vi "Scan TU Number_RegExp.vi"(10 "Pattern In":string) -> (1 "OK?":bool, 3 "TU Number Out":string)   [LabVIEW 2024, in "LVarex.lvlib"]
uses:
  LVarex.lvlib
panel:
  out "First Scan?":bool
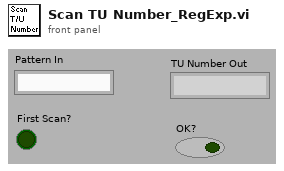
[diagram p1: front panel]
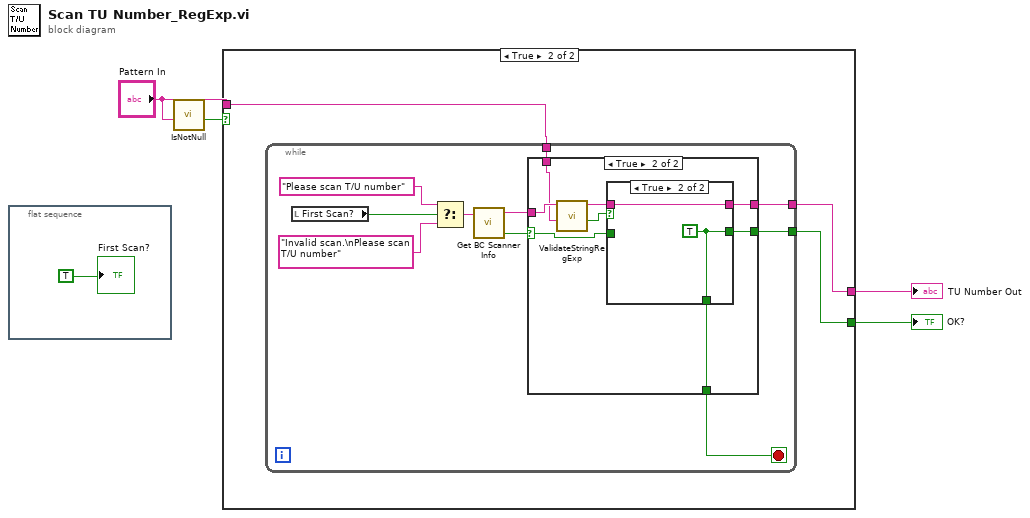
[diagram p0: block diagram]
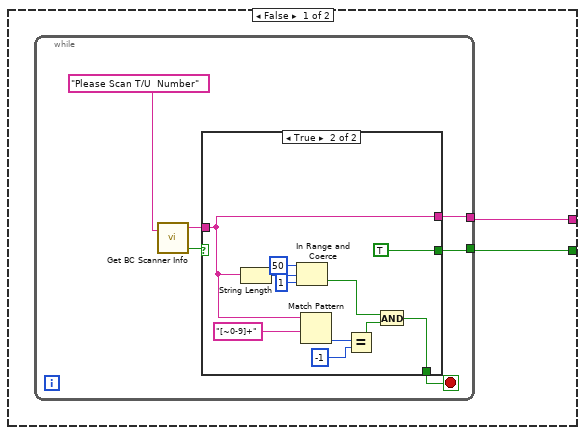
[diagram p2: hidden frame]
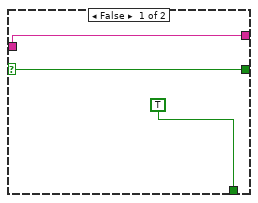
[diagram p3: hidden frame]
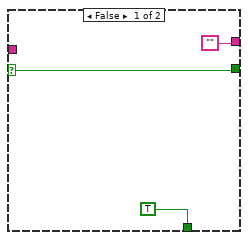
[diagram p4: hidden frame]
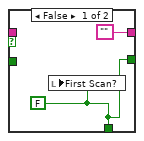
[diagram p5: hidden frame]
diagram:
  n1 = flat-sequence {
    frame #0 {
      "First Scan?" <- TRUE
    }
  }
  n2 = call "IsNotNull.vi"("String In"="Pattern In") -> ("Boolean Out"=w1:bool)  [unwired: 10 in]
  n3 = case shown="True" w1 {
    tunnel: [w7 w30] -> w4
    tunnel: [w6 w29] -> w3
    tunnel: "Pattern In" -> [_ w28]
    frame False {
      n4 = while {
        tunnel: [w11] -> w6
        tunnel: [w10] -> w7
        stop <- w9 stop-if-true
        n5 = call "Get BC Scanner Info.vi"("Prompt"="Please Scan T/U  Number") -> ("Info Out"=w8:string, "OK"=w12:bool)  [unwired: 2 in]
        n6 = case shown="True" w12 {
          selector: w12 -> [w16 _]
          tunnel: [w16 TRUE] -> w11
          tunnel: w8 -> [w15 w23]
          tunnel: [w15 w23] -> w10
          tunnel: [TRUE w17] -> w9
          frame False {
          }
          frame True {
            n7 = String Length(string=w23) -> (length=w26:i32)
            n8 = In Range and Coerce(upper limit=50, x=w26, lower limit=1) -> (In Range?=w18:bool)  [unwired: 1 out]
            n9 = Match Pattern(string=w23, regular expression="[~0-9]+") -> (offset past match=w21:i32)  [unwired: 1 in, 3 out]
            n10 = Equal?(x=w21, y=-1 ("x")) -> (x = y?=w19:bool)
            n11 = And(x=w18, y=w19) -> (x .and. y?=w17:bool)
          }
        }
      }
    }
    frame True {
      n12 = while {
        tunnel: [w34] -> w30
        tunnel: [w33] -> w29
        tunnel: w28 -> [w31]
        stop <- w32 stop-if-true
        n13 = local read "First Scan?"() -> (w38:bool)
        n14 = Select(t="Please scan T/U number", s=w38, f="Invalid scan.\nPlease scan T/U number") -> (s? t:f=w37:string)
        n15 = call "Get BC Scanner Info.vi"("Prompt"=w37) -> ("Info Out"=w36:string, "OK"=w35:bool)  [unwired: 2 in]
        n16 = case shown="True" w35 {
          selector: w35 -> [w41 w50]
          tunnel: w36 -> [_ w46]
          tunnel: ["" w51] -> w34
          tunnel: [w41 w49] -> w33
          tunnel: [TRUE w48] -> w32
          tunnel: w31 -> [_ w45]
          frame False {
          }
          frame True {
            n17 = call "ValidateStringRegExp.vi"("Pattern In"=w45, "String To Match"=w46) -> ("Match Found"=w44:bool, "String Out"=w47:string)  [unwired: 8 in]
            n18 = case shown="True" w44 {
              tunnel: w47 -> [_ w55]
              tunnel: ["" w55] -> w51
              tunnel: w50 -> [_ _]
              tunnel: [w53 w54] -> w49
              tunnel: [w53 w54] -> w48
              frame False {
                w53 = FALSE
                n19 = local write "First Scan?"(w53) -> ()
              }
              frame True {
                w54 = TRUE
              }
            }
          }
        }
      }
    }
  }
  "TU Number Out" <- w4
  "OK?" <- w3
